vi "FF_Wall.vi"(8 "error in (no error)":errorcluster, 9 "WristVelocity":dbl[](array[numeric]), 10 "WristPosition":dbl[](array[numeric]), 11 "Force Field Controller in":refnum<class "ForceField.lvclass">) -> (0 "error out":errorcluster, 1 "ClosestPt":dbl[](array[numeric]), 2 "Force":dbl[](array[numeric]), 3 "Force Field Controller out":refnum<class "ForceField.lvclass">, 4 "ForceComp":dbl[](array[numeric]))   [LabVIEW 2016, in "ForceField.lvclass"]
uses:
  ForceField.lvclass
  TypeDef/TND.ctl
  ForceField.lvclass/ForceField.ctl
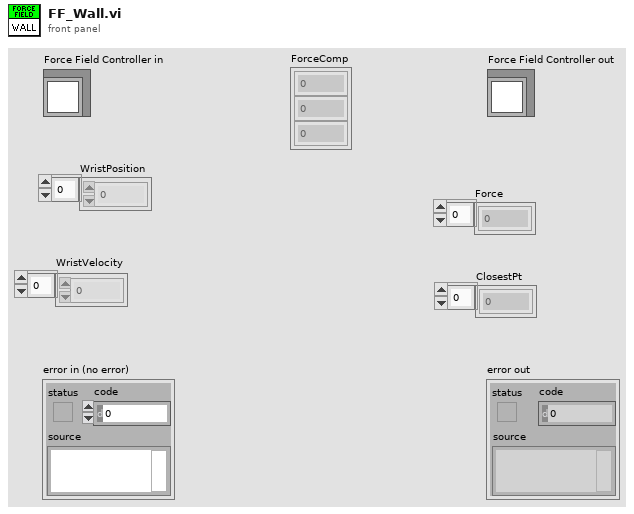
[diagram p1: front panel]
types:
  T1 = typedef "ForceField.lvclass/TND.ctl" = cluster{"Vt":dbl[], "Vn":dbl[], "Dmin":dbl}
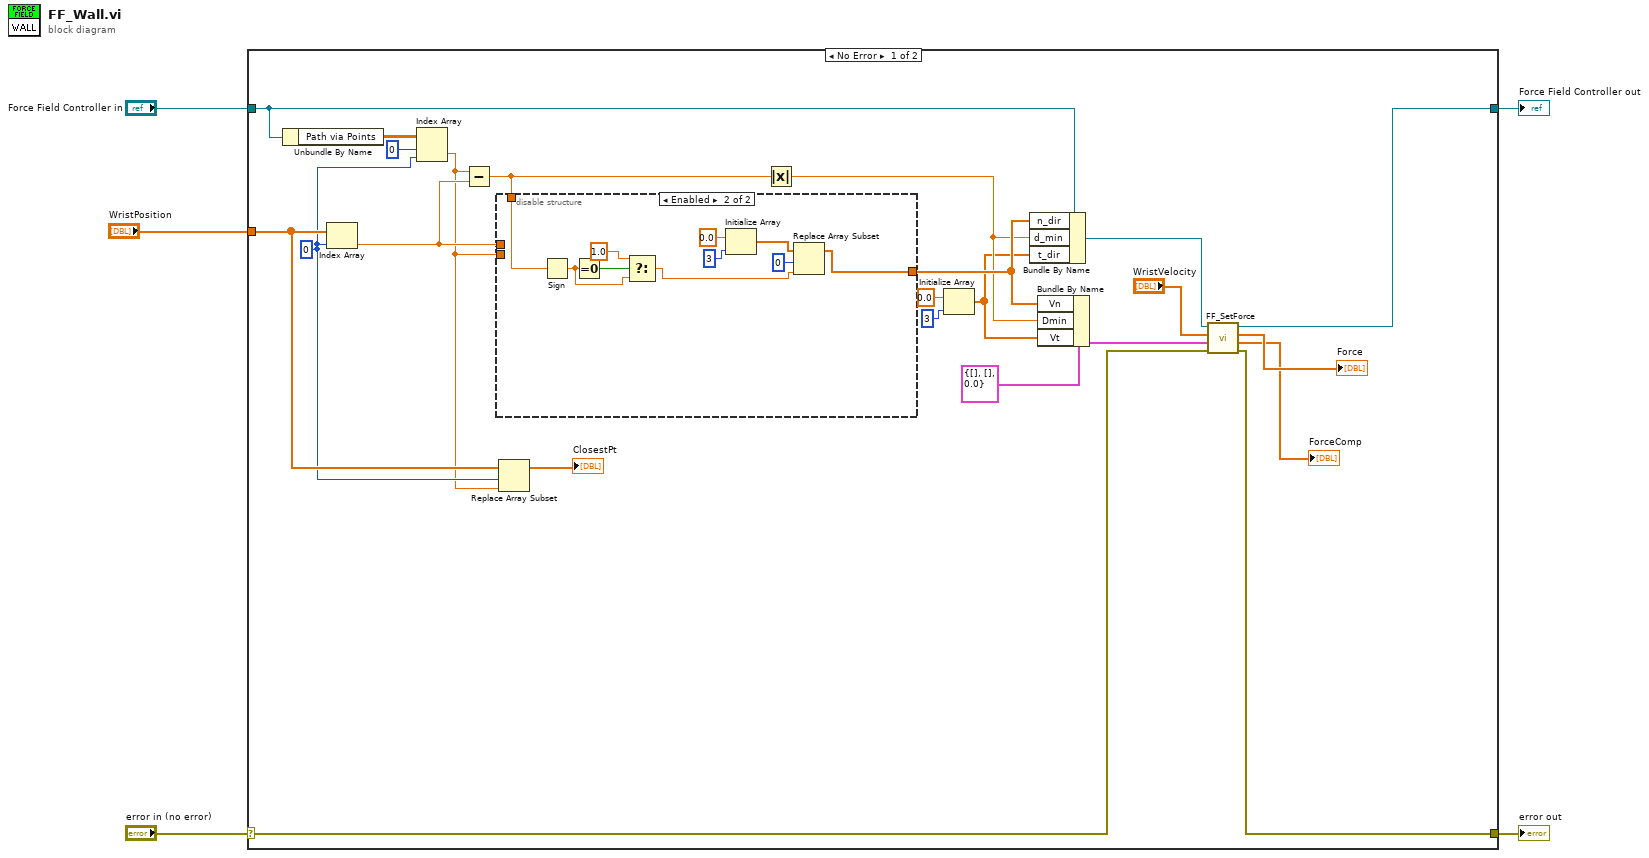
[diagram p0: block diagram]
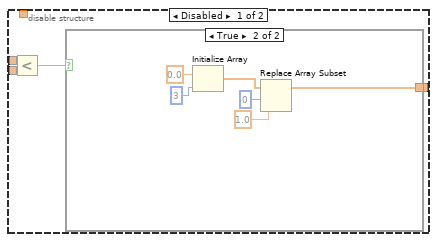
[diagram p2: hidden frame]
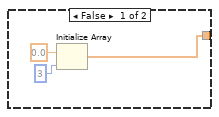
[diagram p3: hidden frame]
diagram:
  n1 = case shown="No Error" "error in (no error)" {
    selector: "error in (no error)" -> [w18 w53]
    tunnel: [w17 w53] -> w4
    tunnel: [w19 w52] -> w2
    tunnel: "Force Field Controller in" -> [w26 w52]
    tunnel: "WristPosition" -> [w15 _]
    frame No Error {
      w14 = 0 ("disabled index (col)")
      n2 = Unbundle By Name(w26) -> ("Path via Points"=w28:dbl[][])
      n3 = Index Array(array=w15, index=w14) -> (element=w25:dbl)
      n4 = Index Array(array=w28, index (row)=0, index (col)=w14) -> (element=w13:dbl)
      n5 = Subtract(x=w13, y=w25) -> (x-y=w16:dbl)
      n6 = disable-structure shown="Enabled" {
        disable-tunnel: [w31 w42] -> w8
        disable-tunnel: w13 -> [w30 _]
        disable-tunnel: w25 -> [w29 _]
        disable-tunnel: w16 -> [_ w51]
        frame Disabled {
          n7 = Less?(x=w29, y=w30) -> (x < y?=w32:bool)
          n8 = case shown="True" w32 {
            tunnel: [w34 w36] -> w31
            frame False {
              n9 = Initialize Array(0.0 ("element"), 3 ("dimension size")) -> (w34:dbl[])
            }
            frame True {
              n10 = Initialize Array(0.0 ("element"), 3 ("dimension size")) -> (w39:dbl[])
              n11 = Replace Array Subset(array=w39, new element=1.0 ("new element/subarray"), index=0) -> (w36:dbl[])
            }
          }
        }
        frame Enabled {
          n12 = Sign(1:w51) -> (0:w49:dbl)
          n13 = Equal To 0?(x=w49) -> (x = 0?=w50:bool)
          n14 = Select(t=1.0, s=w50, f=w49) -> (s? t:f=w43:dbl)
          n15 = Initialize Array(0.0 ("element"), 3 ("dimension size")) -> (w45:dbl[])
          n16 = Replace Array Subset(array=w45, new element=w43, index=0) -> (w42:dbl[])
        }
      }
      n17 = Replace Array Subset(array=w15, new element=w13, index=w14) -> (→"ClosestPt":dbl[])
      n18 = Absolute Value(x=w16) -> (abs(x)=w7:dbl)
      n19 = Initialize Array(0.0 ("element"), 3 ("dimension size")) -> (w6:dbl[])
      n20 = Bundle By Name(cluster=w26, "n_dir"=w8, "d_min"=w7, "t_dir"=w6) -> (w20:refnum<class "ForceField.lvclass">)
      n21 = Bundle By Name(cluster=T1 {"Vt"=[], "Vn"=[], "Dmin"=0.0} ("TND"), "Vn"=w8, "Dmin"=w7, "Vt"=w6) -> (w9:T1)
      n22 = call "FF_SetForce.vi"("error in (no error)"=w18, "TND"=w9, "AnkleVelocity"="WristVelocity", "Force Field Controller in"=w20) -> ("error out"=w17:errorcluster, "ForceNTD"=→"ForceComp":dbl[], "ForceXYZ"=→"Force":dbl[], "Force Field Controller out"=w19:refnum<class "ForceField.lvclass">)  [unwired: 4 in]
    }
    frame Error {
    }
  }
  "error out" <- w4
  "Force Field Controller out" <- w2
